vi "Write Stop Process Ref.vi"(6 "Wash Entry Ref":refnum<vi>, 11 "Car Wash Status View Definition in":refnum<class "Stop Process View Definition.lvclass">) -> (3 "Car Wash Status View Definition out":refnum<class "Stop Process View Definition.lvclass">)   [LabVIEW 2019, in "Stop Process View Definition.lvclass"]
uses:
  <vilib>/gpm_packages/@cs/Car-wash/Source/Stop Process View Definition/Stop Process View Definition.lvclass
  <vilib>/gpm_packages/@cs/Car-wash/Source/Stop Process View Definition/Stop Process View Definition.lvclass/Stop Process View Definition.ctl
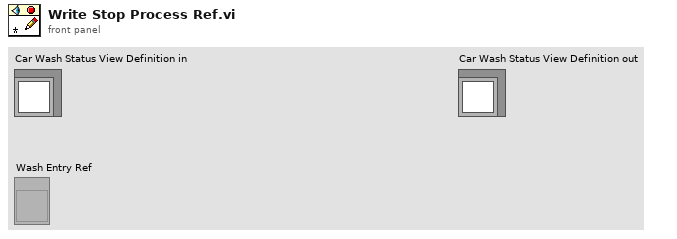
[diagram p1: front panel]
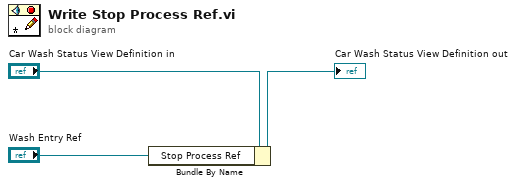
[diagram p0: block diagram]
diagram:
  n1 = Bundle By Name(cluster="Car Wash Status View Definition in", "Stop Process Ref"="Wash Entry Ref") -> (→"Car Wash Status View Definition out":refnum<class "Stop Process View Definition.lvclass">)
